vi "1.2.1.4-Gen RW Idle Case.vi"(0 "Clk":i8) -> (1 "Clk=-1;":i8, 2 "State":T1(ring))   [LabVIEW 2011]
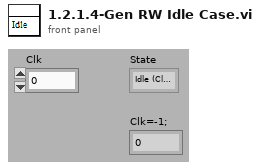
[diagram p1: front panel]
types:
  T1 = enum8{"Idle (Clk=-1)", "Sending(Clk*==Clk+1?Clk=Clk*:;)", "Receiving(Clk*==Clk?Clk++:;)"}
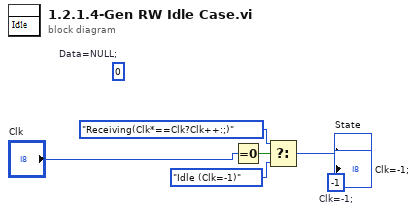
[diagram p0: block diagram]
diagram:
  (unwired) u8 0  # Data=NULL;
  w6 = i8 -1  # Clk=-1;
  n1 = Equal To 0?(x="Clk") -> (x = 0?=w2:bool)
  n2 = Select(t=T1."Receiving(Clk*==Clk?Clk++:;)" ("State"), s=w2, f=T1."Idle (Clk=-1)" ("State")) -> (s? t:f=→"State":T1)
  "Clk=-1;" <- w6
